vi "GenNet Version-Safe Unflatten Variant.vi"(8 "error in":errorcluster, 11 "Flattened Data":string) -> (0 "error out":errorcluster, 3 "Message Data":variant)   [LabVIEW 2014, in "hse-gennet.lvlib"]
doc: "Unflattens a variant from a string. Automatically prepends the correct header if the variant was flattened in another LabVIEW version.\n\n____\nHAMPEL SOFTWARE ENGINEERING v0.7.0 (2018-07-16 18:12)"
uses:
  hse-gennet.lvlib
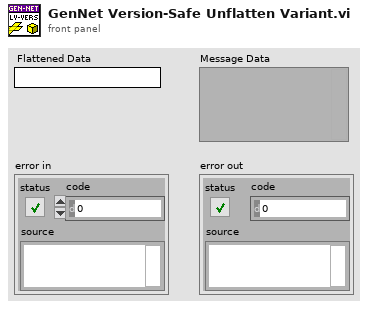
[diagram p1: front panel]
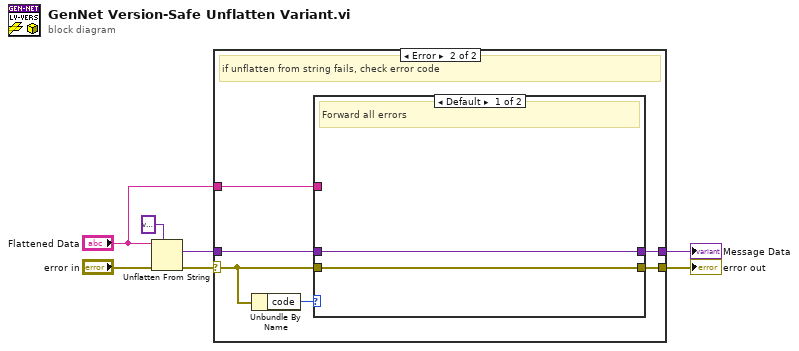
[diagram p0: block diagram]
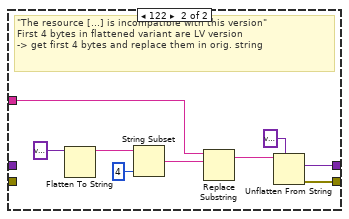
[diagram p3: hidden frame]
diagram:
  n1 = Unflatten From String(type=variant ("Message Data"), binary string="Flattened Data", error in (no error)="error in") -> (value=w6:variant, error out=w4:errorcluster)  [unwired: 2 in, 1 out]
  n2 = case shown="Error" w4 {
    selector: w4 -> [w9 w14]
    tunnel: w6 -> [w8 w12]
    tunnel: [w9 w13] -> w3
    tunnel: [w8 w11] -> w2
    tunnel: "Flattened Data" -> [_ w10]
    frame No Error {
    }
    frame Error {
      # "if unflatten from string fails, check error code"
      n3 = Unbundle By Name(w14) -> ("code"=w15:i32)
      n4 = case shown="Default" w15 {
        tunnel: w14 -> [w17 _]
        tunnel: [w17 w20] -> w13
        tunnel: w12 -> [w16 _]
        tunnel: [w16 w19] -> w11
        tunnel: w10 -> [_ w25]
        frame Default {
          # "Forward all errors"
        }
        frame 122 {
          # "\"The resource [...] is incompatible with this version\"\nFirst 4 bytes in flattened variant are LV version\n-> get first 4 bytes and replace them in orig. string"
          n5 = Flatten To String(anything=variant) -> (data string=w24:string)  [unwired: 3 in, 2 out]
          n6 = String Subset(string=w24, length (rest)=4 ("length (rest)")) -> (substring=w22:string)  [unwired: 1 in]
          n7 = Replace Substring(4:w22, 5:w25) -> (1:w18:string)  [unwired: 2 in, 1 out]
          n8 = Unflatten From String(type=variant ("Message Data"), binary string=w18) -> (value=w19:variant, error out=w20:errorcluster)  [unwired: 3 in, 1 out]
        }
      }
    }
  }
  "Message Data" <- w2
  "error out" <- w3
